vi "Apply TTL Property.vi"(0 "State in":refnum<class "State.lvclass">, 5 "param":string, 7 "value":dbl, 9 "chan":string, 11 "error in (no error)":errorcluster, 12 "TTL name":string) -> (4 "State out":refnum<class "State.lvclass">, 15 "error out":errorcluster)   [LabVIEW 2015, in "State.lvclass"]
uses:
  State.lvclass
  State.lvclass/State.ctl
  Termination/Termination.lvclass/Termination.ctl
  Timeout/Timeout.lvclass/Timeout.ctl
  Termination/Read TTL.vi
  Termination/Write TTL.vi
  Timeout/Read TTL.vi
  Timeout/Write TTL.vi
  TTL VIs/Control Classes/Base Class/TTLController.lvclass
  Termination/Termination.lvclass
  Timeout/Timeout.lvclass
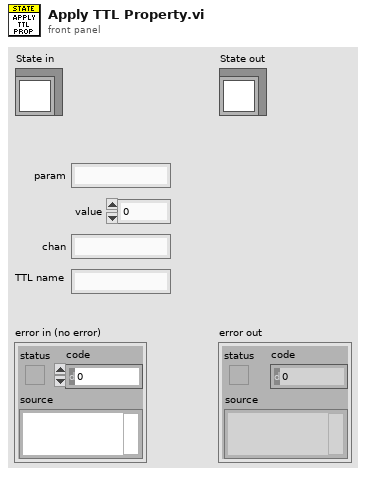
[diagram p1: front panel]
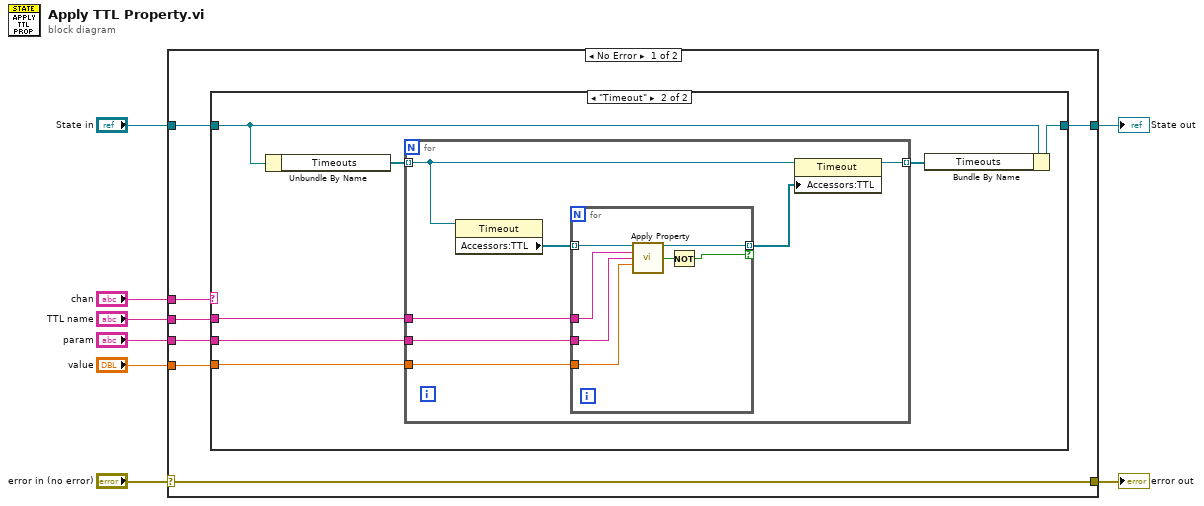
[diagram p0: block diagram]
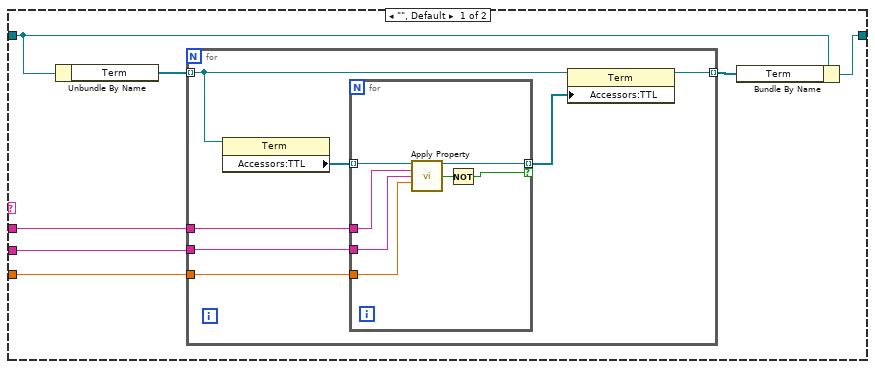
[diagram p2: hidden frame]
diagram:
  n1 = case shown="No Error" "error in (no error)" {
    selector: "error in (no error)" -> [w15 w59]
    tunnel: [w15 w59] -> w7
    tunnel: [w9 w58] -> w5
    tunnel: "State in" -> [w10 w58]
    tunnel: "chan" -> [w14 _]
    tunnel: "TTL name" -> [w13 _]
    tunnel: "param" -> [w12 _]
    tunnel: "value" -> [w11 _]
    frame No Error {
      n2 = case shown="\"Timeout\"" w14 {
        tunnel: [w16 w41] -> w9
        tunnel: w13 -> [w22 w42]
        tunnel: w11 -> [w21 w39]
        tunnel: w12 -> [w19 w37]
        tunnel: w10 -> [w18 w38]
        frame "", Default {
          n3 = Unbundle By Name(w18) -> ("Term"=w20:refnum<class "Termination.lvclass">[])
          n4 = for {
            tunnel: w20 -> [w24] mode=indexing
            tunnel: w22 -> [w29]
            tunnel: w21 -> [w28]
            tunnel: w19 -> [w27]
            tunnel: [w23] -> w17 mode=indexing
            n5 = property class="Term"(reference=w24) -> ("Accessors:TTL"=w26:refnum<class "TTLController.lvclass">[])  [unwired: 1 in, 2 out]
            n6 = for {
              tunnel: w26 -> [w35] mode=indexing
              tunnel: w29 -> [w34]
              tunnel: [w31] -> w25 mode=indexing if=w36
              tunnel: w28 -> [w32]
              tunnel: w27 -> [w33]
              n7 = call "Apply Property.vi"("TTLControl in"=w35, "TTL name"=w34, "param"=w33, "value"=w32) -> ("TTLControl out"=w31:refnum<class "TTLController.lvclass">, "Disabled"=w30:bool)  [unwired: 9 in, 1 out]
              n8 = Not(x=w30) -> (.not. x?=w36:bool)
            }
            n9 = property class="Term"(reference=w24, "Accessors:TTL"=w25) -> (reference out=w23:refnum<class "Termination.lvclass">)  [unwired: 1 in, 1 out]
          }
          n10 = Bundle By Name(cluster=w18, "Term"=w17) -> (w16:refnum<class "State.lvclass">)
        }
        frame "Timeout" {
          n11 = Unbundle By Name(w38) -> ("Timeouts"=w43:refnum<class "Timeout.lvclass">[])
          n12 = for {
            tunnel: w43 -> [w50] mode=indexing
            tunnel: w42 -> [w48]
            tunnel: [w44] -> w40 mode=indexing
            tunnel: w39 -> [w46]
            tunnel: w37 -> [w47]
            n13 = property class="Timeout"(reference=w50) -> ("Accessors:TTL"=w45:refnum<class "TTLController.lvclass">[])  [unwired: 1 in, 2 out]
            n14 = for {
              tunnel: w45 -> [w56] mode=indexing
              tunnel: w48 -> [w55]
              tunnel: [w52] -> w49 mode=indexing if=w57
              tunnel: w46 -> [w53]
              tunnel: w47 -> [w54]
              n15 = call "Apply Property.vi"("TTLControl in"=w56, "TTL name"=w55, "param"=w54, "value"=w53) -> ("TTLControl out"=w52:refnum<class "TTLController.lvclass">, "Disabled"=w51:bool)  [unwired: 9 in, 1 out]
              n16 = Not(x=w51) -> (.not. x?=w57:bool)
            }
            n17 = property class="Timeout"(reference=w50, "Accessors:TTL"=w49) -> (reference out=w44:refnum<class "Timeout.lvclass">)  [unwired: 1 in, 1 out]
          }
          n18 = Bundle By Name(cluster=w38, "Timeouts"=w40) -> (w41:refnum<class "State.lvclass">)
        }
      }
    }
    frame Error {
    }
  }
  "error out" <- w7
  "State out" <- w5
